vi "Init.vi"(8 "error in (no error)":errorcluster, 11 "MXN Actor in":refnum<class "MXN Actor.lvclass">) -> (0 "error out":errorcluster, 3 "MXN Actor out":refnum<class "MXN Actor.lvclass">)   [LabVIEW 2019, in "MXN Actor.lvlib" / "MXN Actor.lvclass"]
uses:
  MXN Actor.lvclass
  MXN Actor.lvclass/MXN Actor.ctl
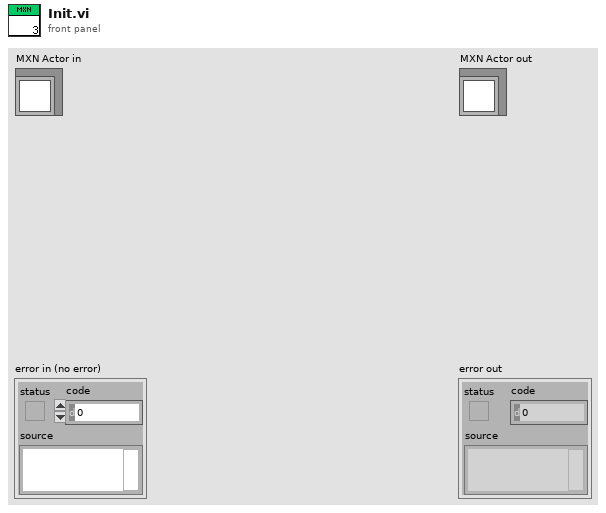
[diagram p1: front panel]
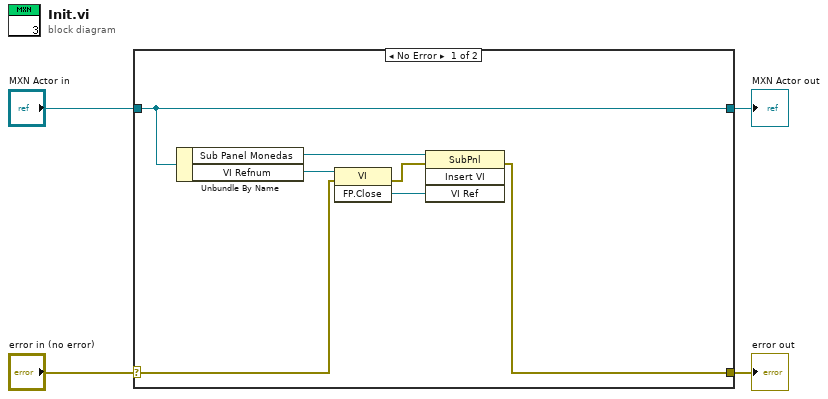
[diagram p0: block diagram]
diagram:
  n1 = case shown="No Error" "error in (no error)" {
    selector: "error in (no error)" -> [w6 w13]
    tunnel: [w5 w13] -> w3
    tunnel: [w11 w12] -> w1
    tunnel: "MXN Actor in" -> [w11 w12]
    frame No Error {
      n2 = Unbundle By Name(w11) -> ("Sub Panel Monedas"=w10:refnum<vi>, "VI Refnum"=w9:refnum<vi>)
      n3 = invoke class="VI" method="FP.Close"(reference=w9, error in=w6) -> (reference out=w8:refnum<vi>, error out=w7:errorcluster)  [unwired: 1 in, 1 out]
      n4 = invoke class="SubPnl" method="Insert VI"(reference=w10, error in=w7, "VI Ref"=w8) -> (error out=w5:errorcluster)  [unwired: 1 in, 3 out]
    }
    frame Error {
    }
  }
  "error out" <- w3
  "MXN Actor out" <- w1
